vi "Write configuration.vi"(8 "error in":errorcluster, 10 "configuration":refnum<class "NISE_CEF_serializable configuration.lvclass">, 11 "Cfg Channel in":refnum<class "Cfg Channel.lvclass">) -> (0 "error out":errorcluster, 3 "Cfg Channel out":refnum<class "Cfg Channel.lvclass">)   [LabVIEW 2013, in "Cfg Channel.lvclass"]
uses:
  Cfg Channel.lvclass
  CEF_TreeControl/serializable configuration/NISE_CEF_serializable configuration.lvclass
  chcfg/channel config object.lvclass
  Cfg Channel.lvclass/Cfg Channel.ctl
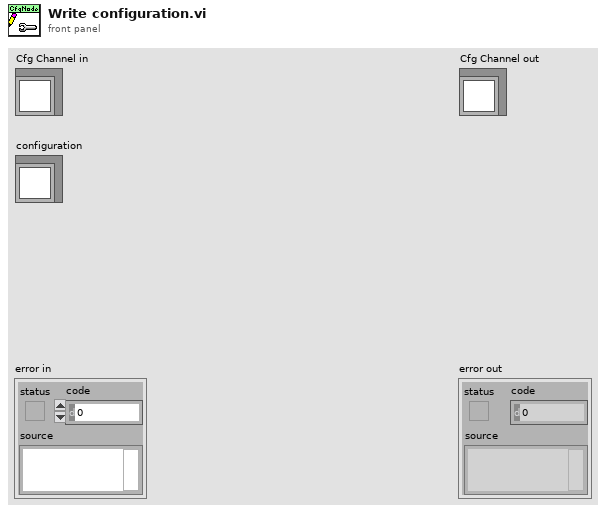
[diagram p1: front panel]
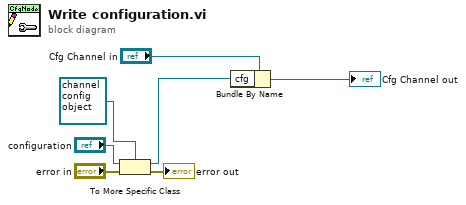
[diagram p0: block diagram]
diagram:
  n1 = To More Specific Class(target class=refnum<class "channel config object.lvclass"> refnum ("channel config object.lvclass"), reference="configuration", error in="error in") -> (specific class reference=w2:refnum<class "channel config object.lvclass">, error out=→"error out":errorcluster)
  n2 = Bundle By Name(cluster="Cfg Channel in", "cfg"=w2) -> (→"Cfg Channel out":refnum<class "Cfg Channel.lvclass">)
